vi "WSVCAP SHL Host LL Manager.vi"(1 "FPGA Resource (Init Only)":tag, 11 "error in (no error)":errorcluster, 12 "Simulate FPGA (Init Only)":bool=TRUE, 13 "Operation":T2) -> (15 "error out":errorcluster)   [LabVIEW 2012]
uses:
  Type Defs/WSVCAP SHL Manager Operation Enum.ctl
  Type Defs/WSVCAP SHL System Cluster.ctl
  Type Defs/WSVCAP SHL Top Level Control Operation Enum.ctl
  <vilib>/FPGAPlugInAG/PXI-7813R/niLvFpga_Open_PXI-7813R.vi
  <vilib>/FPGAPlugInAG/PXI-7813R/niLvFpga_Reset_PXI-7813R.vi
  <vilib>/FPGAPlugInAG/PXI-7813R/niLvFpga_Run_PXI-7813R.vi
  <vilib>/FPGAPlugInAG/PXI-7813R/niLvFpga_Abort_PXI-7813R.vi
  <vilib>/FPGAPlugInAG/PXI-7813R/niLvFpga_Close_PXI-7813R.vi
  <vilib>/rvi/interface/nirviOpenFPGA/nirviOpenFPGA.xnode
  FPGA Bitfiles/WSVCAPShell_WiSpryFPGA1_WSVCAPSHLFPGATLT_8e7AIp0f5+c.lvbitx
  <vilib>/rvi/interface/nirviMethod/nirviMethod.xnode
  <vilib>/rvi/interface/nirviCloseFPGA/nirviCloseFPGA.xnode
panel:
  out "System":T1
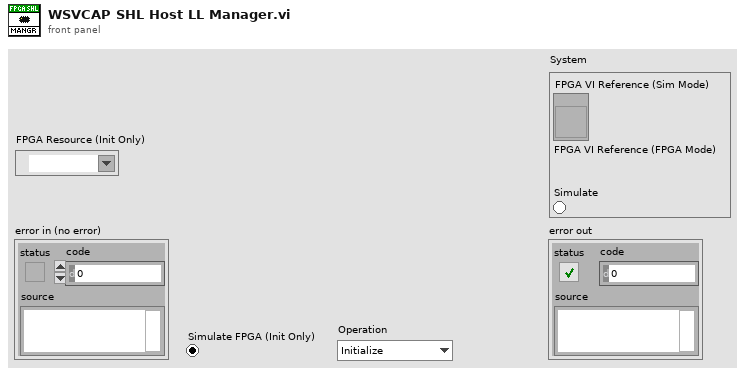
[diagram p1: front panel]
types:
  T1 = typedef "WSVCAP SHL System Cluster.ctl" = cluster{"FPGA VI Reference (Sim Mode)":refnum<vi>, "FPGA VI Reference (FPGA Mode)":refnum<k20>, "Simulate":bool}
  T2 = typedef "WSVCAP SHL Manager Operation Enum.ctl" = enum16{"Initialize", "Close"}
  T3 = typedef "WSVCAP SHL Top Level Control Operation Enum.ctl" = enum16{"Initialize", "Set Control", "Read Control", "Close"}
  T4 = enum32{"Invalid", "Standard", "Closed", "Hidden", "Minimized", "Maximized"}
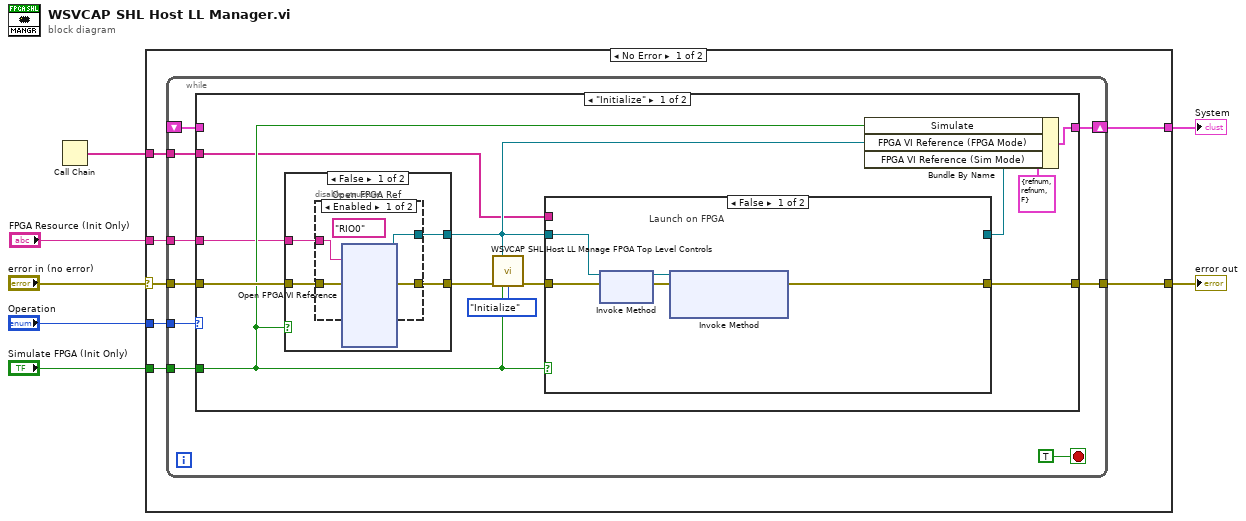
[diagram p0: block diagram]
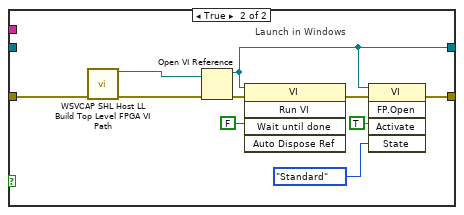
[diagram p4: hidden frame]
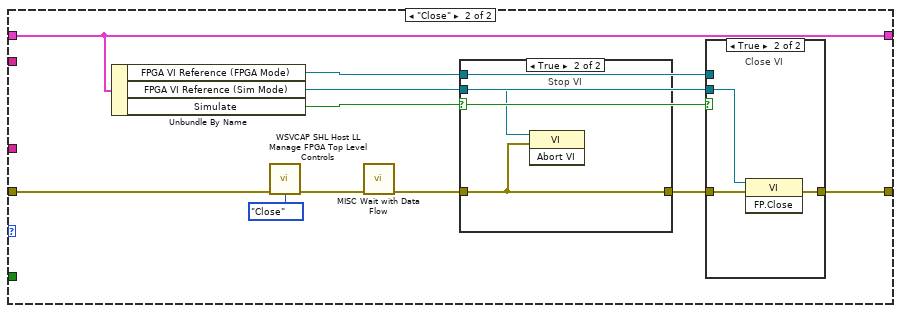
[diagram p5: hidden frame]
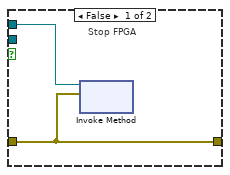
[diagram p6: hidden frame]
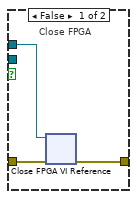
[diagram p7: hidden frame]
diagram:
  n1 = Call Chain() -> (call chain=w1:string[])
  n2 = case shown="No Error" "error in (no error)" {
    selector: "error in (no error)" -> [w14 _]
    tunnel: [w13 _] -> w6
    tunnel: "Operation" -> [w12 _]
    tunnel: "Simulate FPGA (Init Only)" -> [w11 _]
    tunnel: [w10 _] -> w3
    tunnel: "FPGA Resource (Init Only)" -> [w9 _]
    tunnel: w1 -> [w8 _]
    frame No Error {
      n3 = while {
        tunnel: w14 -> [w23]
        tunnel: [w22] -> w13
        tunnel: w12 -> [w20]
        tunnel: w11 -> [w19]
        shift-right: [w18] -> w10
        shift-left: _ -> [w17]
        tunnel: w9 -> [w16]
        tunnel: w8 -> [w15]
        stop <- TRUE stop-if-true
        n4 = case shown="\"Initialize\"" w20 {
          tunnel: w23 -> [w33 w68]
          tunnel: [w25 w67] -> w22
          tunnel: w19 -> [w27 _]
          tunnel: [w30 w69] -> w18
          tunnel: w17 -> [_ w69]
          tunnel: w16 -> [w26 _]
          tunnel: w15 -> [w24 _]
          frame "Initialize" {
            n5 = case shown="False" w27 {
              tunnel: [w39 w45] -> w35
              tunnel: w33 -> [w38 w45]
              tunnel: [w37 _] -> w29
              tunnel: w26 -> [w36 _]
              frame False {
                # "Open FPGA Ref"
                n6 = disable-structure shown="Enabled" {
                  disable-tunnel: w38 -> [w43 w44]
                  disable-tunnel: [w42 w44] -> w39
                  disable-tunnel: [w41 _] -> w37
                  disable-tunnel: w36 -> [w40 _]
                  frame Enabled {
                    (unwired) tag "RIO0" ("resource name")
                    n7 = xnode "Open FPGA VI Reference"("error in"=w43, "resource name"=w40) -> ("FPGA VI Reference Out"=w41:refnum<k20>, "error out"=w42:errorcluster)
                  }
                  frame Disabled {
                  }
                }
              }
              frame True {
                # "Simulate FPGA"
              }
            }
            n8 = call "WSVCAP SHL Host LL Manage FPGA Top Level Controls.vi"("FPGA VI Reference (Init Only)"=w29, "error in (no error)"=w35, "Simulate FPGA (Init Only)"=w27, "Operation"=WSVCAP_SHL_Top_Level_Control_Operation_Enum."Initialize") -> ("error out"=w32:errorcluster)  [unwired: 10 in, 1 out]
            n9 = case shown="False" w27 {
              tunnel: w32 -> [w49 w53]
              tunnel: [w48 w56] -> w25
              tunnel: w29 -> [w46 _]
              tunnel: [_ w57] -> w28
              tunnel: w24 -> [_ _]
              frame False {
                # "Launch on FPGA"
                n10 = xnode "Invoke Method"("FPGA VI Reference In"=w46, "error in"=w49) -> ("FPGA VI Reference Out"=w47:refnum<k20>, "error out"=w50:errorcluster)
                n11 = xnode "Invoke Method"("FPGA VI Reference In"=w47, "error in"=w50) -> ("error out"=w48:errorcluster)  [unwired: 1 in, 1 out]
              }
              frame True {
                # "Launch in Windows"
                n12 = call "WSVCAP SHL Host LL Build Top Level FPGA VI Path.vi"("Error In (no error)"=w53) -> ("Top Level FPGA VI Path"=w51:path, "Error Out"=w52:errorcluster)  [unwired: 13 in]
                n13 = Open VI Reference(vi path=w51, error in (no error)=w52) -> (vi reference=w57:refnum<vi>, error out=w60:errorcluster)  [unwired: 4 in]
                n14 = invoke class="VI" method="Run VI"(reference=w57, error in=w60, "Wait until done"=FALSE ("Wait Until Done")) -> (error out=w58:errorcluster)  [unwired: 2 in, 4 out]
                n15 = invoke class="VI" method="FP.Open"(reference=w57, error in=w58, "Activate"=TRUE ("Activate?"), "State"=T4."Standard" ("Front Panel Window:State")) -> (error out=w56:errorcluster)  [unwired: 1 in, 4 out]
              }
            }
            n16 = Bundle By Name(cluster=T1 {"FPGA VI Reference (Sim Mode)"=refnum, "FPGA VI Reference (FPGA Mode)"=refnum, "Simulate"=FALSE} ("System"), "Simulate"=w27, "FPGA VI Reference (FPGA Mode)"=w29, "FPGA VI Reference (Sim Mode)"=w28) -> (w30:T1)
          }
          frame "Close" {
            n17 = Unbundle By Name(w69) -> ("FPGA VI Reference (FPGA Mode)"=w65:refnum<k20>, "FPGA VI Reference (Sim Mode)"=w63:refnum<vi>, "Simulate"=w66:bool)
            n18 = call "WSVCAP SHL Host LL Manage FPGA Top Level Controls.vi"("error in (no error)"=w68, "Operation"=WSVCAP_SHL_Top_Level_Control_Operation_Enum."Close") -> ("error out"=w62:errorcluster)  [unwired: 12 in, 1 out]
            n19 = call "MISC Wait with Data Flow.vi"("Error In (no error)"=w62) -> ("Error Out"=w61:errorcluster)  [unwired: 8 in, 2 out]
            n20 = case shown="True" w66 {
              tunnel: w65 -> [w72 _]
              tunnel: w61 -> [w71 w73]
              tunnel: [w71 w73] -> w64
              tunnel: w63 -> [_ w74]
              frame False {
                # "Stop FPGA"
                n21 = xnode "Invoke Method"("FPGA VI Reference In"=w72, "error in"=w71) -> ()  [unwired: 2 out]
              }
              frame True {
                # "Stop VI"
                n22 = invoke class="VI" method="Abort VI"(reference=w74, error in=w73) -> ()  [unwired: 1 in, 3 out]
              }
            }
            n23 = case shown="True" w66 {
              tunnel: w64 -> [w77 w80]
              tunnel: w65 -> [w76 _]
              tunnel: [w75 w79] -> w67
              tunnel: w63 -> [_ w78]
              frame False {
                # "Close FPGA"
                n24 = xnode "Close FPGA VI Reference"("FPGA VI Reference In"=w76, "error in"=w77) -> ("error out"=w75:errorcluster)
              }
              frame True {
                # "Close VI"
                n25 = invoke class="VI" method="FP.Close"(reference=w78, error in=w80) -> (error out=w79:errorcluster)  [unwired: 1 in, 2 out]
              }
            }
          }
        }
      }
    }
    frame Error {
    }
  }
  "error out" <- w6
  "System" <- w3
